vi "GraphScale.vi"(8 "error in":errorcluster, 11 "Gen Refnum":refnum<vi>) -> (0 "error out":errorcluster, 3 "GraphScale out":refnum<class "GraphScale.lvclass">)   [LabVIEW 2014, in "GraphScale.lvclass"]
uses:
  GraphScale.lvclass
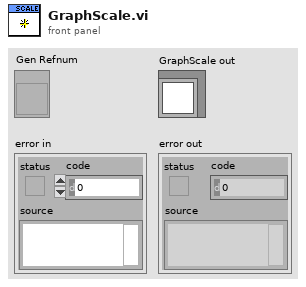
[diagram p1: front panel]
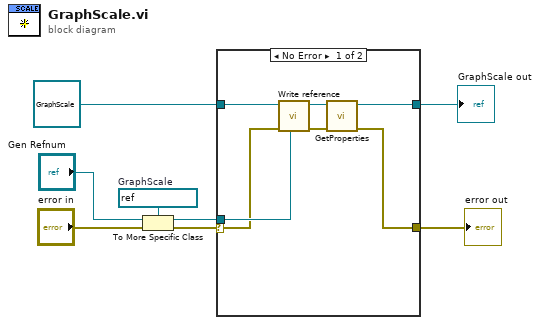
[diagram p0: block diagram]
diagram:
  w6 = refnum<vi> refnum  # GraphScale
  n1 = To More Specific Class(target class=w6, reference="Gen Refnum", error in="error in") -> (specific class reference=w4:refnum<vi>, error out=w5:errorcluster)
  n2 = case shown="No Error" w5 {
    selector: w5 -> [w13 w17]
    tunnel: w4 -> [w14 _]
    tunnel: refnum<class "GraphScale.lvclass"> refnum ("Scale in") -> [w15 w16]
    tunnel: [w9 w17] -> w1
    tunnel: [w11 w16] -> w2
    frame No Error {
      n3 = call-dynamic "Write reference.vi"("reference"=w14, "error in"=w13, "GObject in"=w15) -> ("error out"=w10:errorcluster, "GObject out"=w12:refnum<class "GraphScale.lvclass">)  [unwired: 5 in]
      n4 = call-dynamic "GetProperties.vi"("error in"=w10, "GraphScale in"=w12) -> ("error out"=w9:errorcluster, "GraphScale out"=w11:refnum<class "GraphScale.lvclass">)  [unwired: 8 in]
    }
    frame Error {
    }
  }
  "error out" <- w1
  "GraphScale out" <- w2
